vi "getPayloadRequirement.vi"(11 "PUBLISH in":refnum<class "PUBLISH.lvclass">) -> (2 "Requirement":T1, 3 "PUBLISH out":refnum<class "PUBLISH.lvclass">)   [LabVIEW 2013, in "MQTT_Control_Packets.lvlib" / "PUBLISH.lvclass"]
uses:
  PUBLISH.lvclass
  ControlPacket/Requirement -- enum.ctl
  ControlPacket/ControlPacket.lvclass
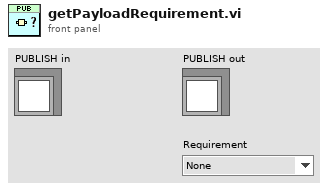
[diagram p1: front panel]
types:
  T1 = typedef "MQTT_Control_Packets.lvlib/ControlPacket.lvclass/Requirement -- enum.ctl" = enum16{"None", "Optional", "Required"}
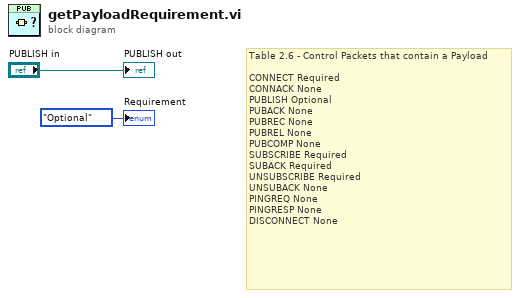
[diagram p0: block diagram]
diagram:
  # "Table 2.6 - Control Packets that contain a Payload\n\nCONNECT Required\nCONNACK None\nPUBLISH Optional\nPUBACK None\nPUBREC None\nPUBREL None\nPUBCOMP None\nSUBSCRIBE Required\nSUBACK Required\nUNSUBSCRIBE Required\nUNSUBACK None\nPINGREQ None\nPINGRESP None\nDISCONNECT None"
  "PUBLISH out" <- "PUBLISH in"
  "Requirement" <- Requirement_--_enum."Optional" ("Requirement")
